vi "OP50B_Data.vi"() -> (0 "OP50B_011_BIC":T1)   [LabVIEW 2020]
uses:
  Controls/OP50B_DataCluster.ctl
panel:
  out "[BIC_MIN]":dbl
  out "[BIC]":dbl
  out "[BIC_MAX]":dbl
  out "[ALPHA0_MIN]":dbl
  out "[ALPHA0]":dbl
  out "[ALPHA0_MAX]":dbl
  out "[ALPHA2_MIN]":dbl
  out "[ALPHA2]":dbl
  out "[ALPHA2_MAX]":dbl
  out "[CT]":dbl
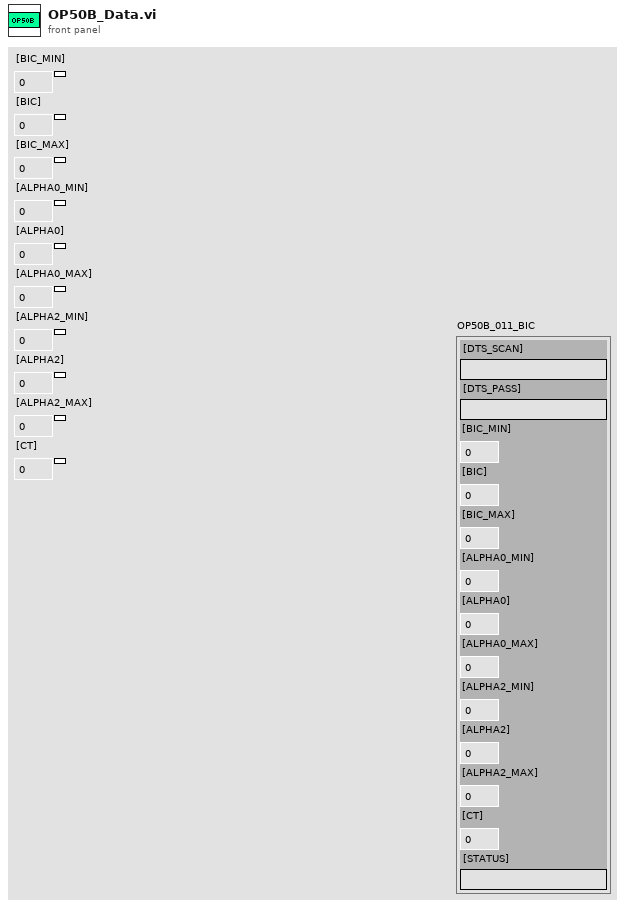
[diagram p1: front panel]
types:
  T1 = typedef "OP50B_DataCluster.ctl" = cluster{"[DTS_SCAN]":string, "[DTS_PASS]":string, "[BIC_MIN]":dbl, "[BIC]":dbl, "[BIC_MAX]":dbl, "[ALPHA0_MIN]":dbl, "[ALPHA0]":dbl, "[ALPHA0_MAX]":dbl, "[ALPHA2_MIN]":dbl, "[ALPHA2]":dbl, "[ALPHA2_MAX]":dbl, "[CT]":dbl, "[STATUS]":string}
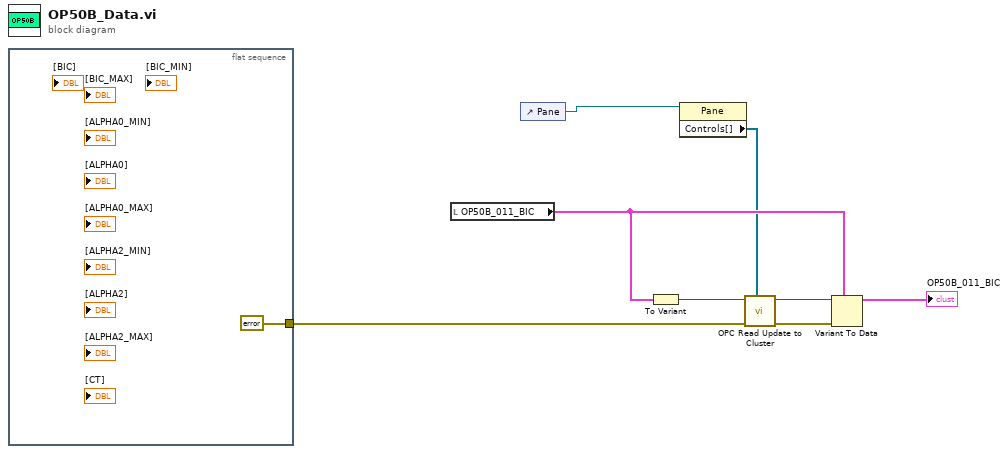
[diagram p0: block diagram]
diagram:
  n1 = flat-sequence {
    tunnel: [errorcluster {"status"=FALSE, "code"=0, "source"=""} ("error in (no error)")] -> w3
    frame #0 {
    }
  }
  n2 = local read "OP50B_011_BIC"() -> (w5:T1)
  n3 = control-ref of="Pane"() -> (w2:refnum<vi>)
  n4 = To Variant(anything=w5) -> (Variant=w6:variant)
  n5 = property class="Pane"(reference=w2) -> ("Controls[]"=w1:refnum<vi>[])  [unwired: 1 in, 2 out]
  n6 = call "OPC Read Update to Cluster.vi"("Controls[]"=w1, "error in (no error)"=w3, "Variant in"=w6) -> ("error out"=w7:errorcluster, "Variant out"=w8:variant)  [unwired: 7 in]
  n7 = Variant To Data(error in=w7, type=w5, Variant=w8) -> (data=→"OP50B_011_BIC":T1)  [unwired: 1 out]
